vi "InitMap.vi"(8 "error in (no error)":errorcluster, 10 "ImagePoll":dbl, 11 "Camera Info":T1) -> (0 "error out":errorcluster, 3 "map out":T2)   [LabVIEW 2017, in "IrAcquisition.lvlib"]
uses:
  <vilib>/addons/InsightCM/Devices/Shared/Ir/IrAcquisition/IrAcquisition.lvlib
  <vilib>/addons/PointValueMap/controls/PointMap.ctl
  <vilib>/addons/InsightCM/Devices/Shared/Ir/IrManageCameras/controls/camera.ctl
  <vilib>/addons/PointValueMap/subVIs/Point_Write_double.vi
  <vilib>/addons/PointValueMap/subVIs/Point_Write_string.vi
  <vilib>/addons/PointValueMap/PointValueMap.lvlib
  <vilib>/addons/InsightCM/Devices/Shared/Ir/IrManageCameras/IrManageCameras.lvlib
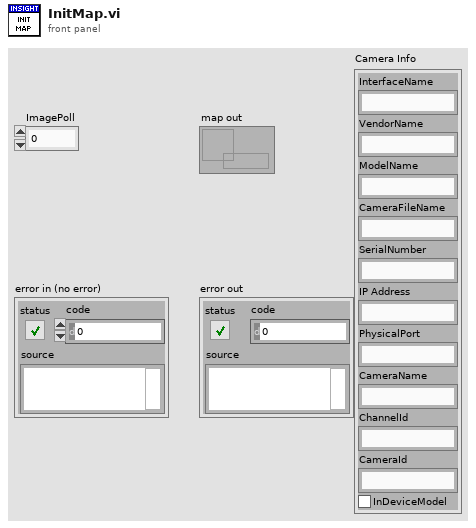
[diagram p1: front panel]
types:
  T1 = typedef "IrManageCameras.lvlib/camera.ctl" = cluster{"InterfaceName":string, "VendorName":string, "ModelName":string, "CameraFileName":string, "SerialNumber":string, "IP Address":string, "PhysicalPort":string, "CameraName":string, "ChannelId":string, "CameraId":string, "InDeviceModel":bool}
  T2 = typedef "PointValueMap.lvlib/PointMap.ctl" = refnum<data-value>
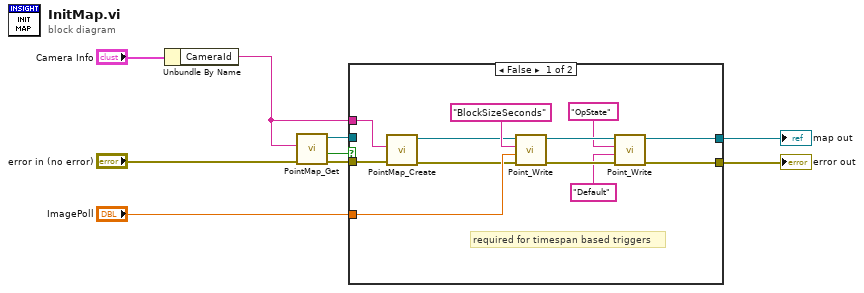
[diagram p0: block diagram]
diagram:
  n1 = Unbundle By Name("Camera Info") -> ("CameraId"=w4:string)
  n2 = call <vilib>:"PointMap_Get.vi"("error in (no error)"="error in (no error)", "Name"=w4) -> ("error out"=w9:errorcluster, "Found?"=w6:bool, "Map Out"=w7:T2)  [unwired: 7 in]
  n3 = case shown="False" w6 {
    tunnel: [w11 w23] -> w2
    tunnel: w7 -> [_ w23]
    tunnel: w4 -> [w21 _]
    tunnel: w9 -> [w20 w22]
    tunnel: [w12 w22] -> w1
    tunnel: "ImagePoll" -> [w14 _]
    frame False {
      # "required for timespan based triggers"
      n4 = call <vilib>:"PointMap_Create.vi"("error in (no error)"=w20, "Name"=w21) -> ("error out"=w13:errorcluster, "Map Out"=w10:T2)  [unwired: 8 in]
      n5 = call-poly <vilib>:"Point_Write.vi"("Error In"=w13, "Value"=w14, "Tag"="BlockSizeSeconds", "Map"=w10) -> ("Error Out"=w19:errorcluster, "Map Out"=w18:T2)  [unwired: 6 in]
      n6 = call-poly <vilib>:"Point_Write.vi"("Error In"=w19, "Value"="Default", "Tag"="OpState", "Map"=w18) -> ("Error Out"=w12:errorcluster, "Map Out"=w11:T2)  [unwired: 6 in]
    }
    frame True {
    }
  }
  "error out" <- w1
  "map out" <- w2
